vi "DeCoF close connection.vi"(4 "error in (no error)":errorcluster, 7 "Connection ID in":T1) -> (0 "error out":errorcluster, 3 "Conncection ID out":T1)   [LabVIEW 2013]
doc: "Closes the connection to the remote device."
uses:
  subVIs/DeCoF connection.ctl
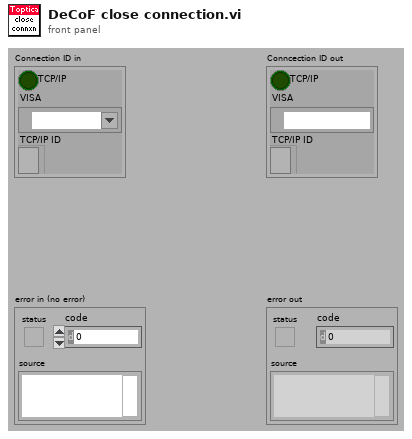
[diagram p1: front panel]
types:
  T1 = typedef "DeCoF connection.ctl" = cluster{"TCP/IP":bool, "VISA":refnum<visa-resource-name>, "TCP/IP ID":refnum<k5>}
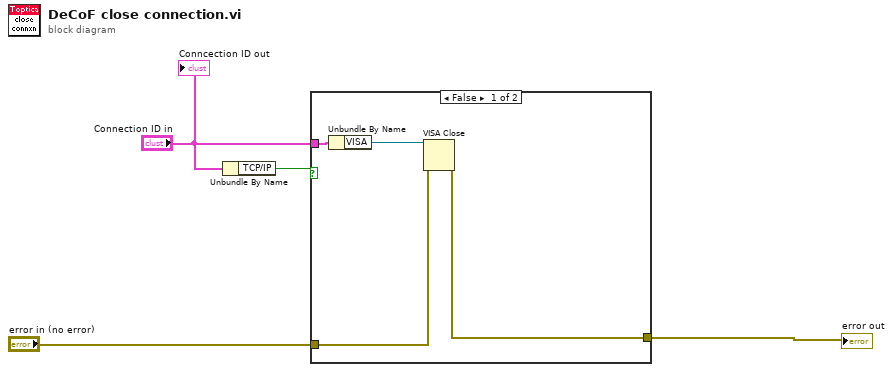
[diagram p0: block diagram]
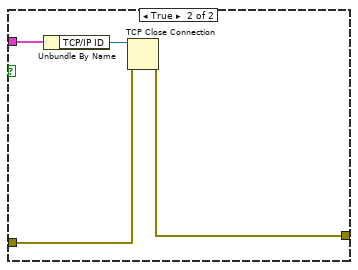
[diagram p2: hidden frame]
diagram:
  n1 = Unbundle By Name("Connection ID in") -> ("TCP/IP"=w1:bool)
  n2 = case shown="False" w1 {
    tunnel: "Connection ID in" -> [w6 w10]
    tunnel: "error in (no error)" -> [w8 w12]
    tunnel: [w7 w11] -> w3
    frame False {
      n3 = Unbundle By Name(w6) -> ("VISA"=w5:refnum<visa-resource-name>)
      n4 = VISA Close(VISA resource name=w5, error in (no error)=w8) -> (error out=w7:errorcluster)
    }
    frame True {
      n5 = Unbundle By Name(w10) -> ("TCP/IP ID"=w9:refnum<k5>)
      n6 = TCP Close Connection(connection ID=w9, error in (no error)=w12) -> (error out=w11:errorcluster)  [unwired: 1 in, 1 out]
    }
  }
  "error out" <- w3
  "Conncection ID out" <- "Connection ID in"
